vi "Align Trajectory.vi"(4 "Force alignemnt":bool=TRUE, 6 "Indicator":refnum<vi>, 7 "Calibration":T1, 8 "error in":errorcluster, 9 "Tip Coordinates":refnum<vi>, 10 "Target Coordinates":refnum<vi>, 11 "Manipulator Interface":T2) -> (0 "error out":errorcluster, 2 "Error":bool)   [LabVIEW 2012, in "Targeting Unit.lvlib"]
uses:
  Targeting Unit.lvlib
  <vilib>/Analysis/Matrix/Datatypes/RealMatrix.ctl
  <vilib>/Analysis/Matrix/NI_Matrix.lvlib
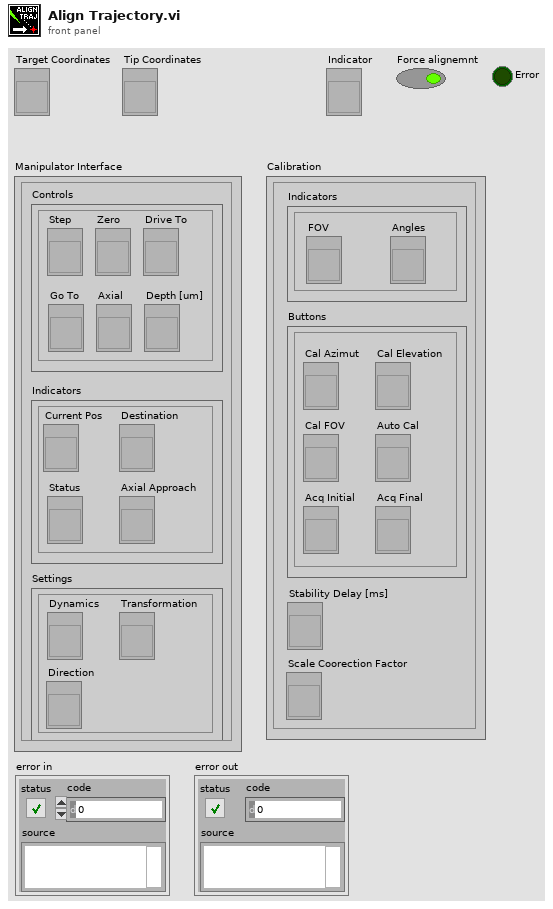
[diagram p1: front panel]
types:
  T1 = cluster{"Indicators":cluster{"FOV":refnum<vi>, "Angles":refnum<vi>}, "Buttons":cluster{"Cal FOV":refnum<vi>, "Cal Azimut":refnum<vi>, "Cal Elevation":refnum<vi>, "Auto Cal":refnum<vi>, "Acq Initial":refnum<vi>, "Acq Final":refnum<vi>}, "Stability Delay [ms]":refnum<vi>, "Scale Coorection Factor":refnum<vi>}
  T2 = cluster{"Indicators":cluster{"Current Pos":refnum<vi>, "Destination":refnum<vi>, "Status":refnum<vi>, "Axial Approach":refnum<vi>}, "Settings":cluster{"Dynamics":refnum<vi>, "Transformation":refnum<vi>, "Direction":refnum<vi>}, "Controls":cluster{"Zero":refnum<vi>, "Step":refnum<vi>, "Drive To":refnum<vi>, "Go To":refnum<vi>, "Axial":refnum<vi>, "Depth [um]":refnum<vi>}}
  T3 = cluster{"X [um]":dbl, "Y [um]":dbl, "Z [um]":dbl}
  T4 = typedef "NI_Matrix.lvlib/RealMatrix.ctl" = dbl[][]
  T5 = cluster{"Step length [um]":dbl, "Interstep Interval [ms]":u32, "Initial Speed [um/s]":dbl, "Max Speed [um/s]":dbl, "Acceleration [um/s^2]":dbl, "Max Depth [um]":dbl, "Max Penetration [um]":dbl}
  T6 = cluster{"X [um]":bool, "Y [um]":bool, "Z [um]":bool}
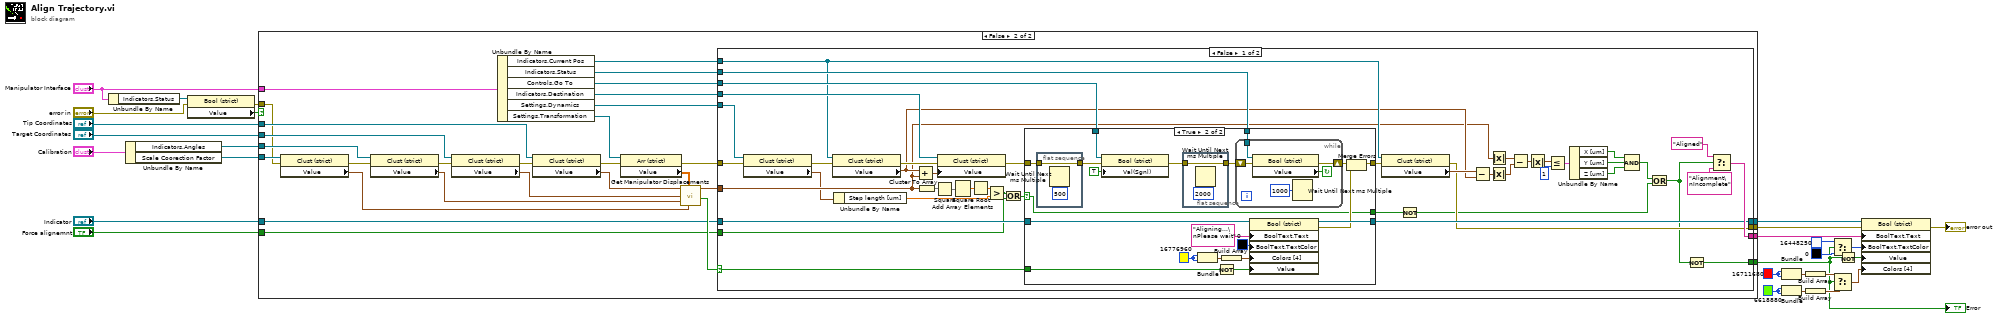
[diagram p0: block diagram]
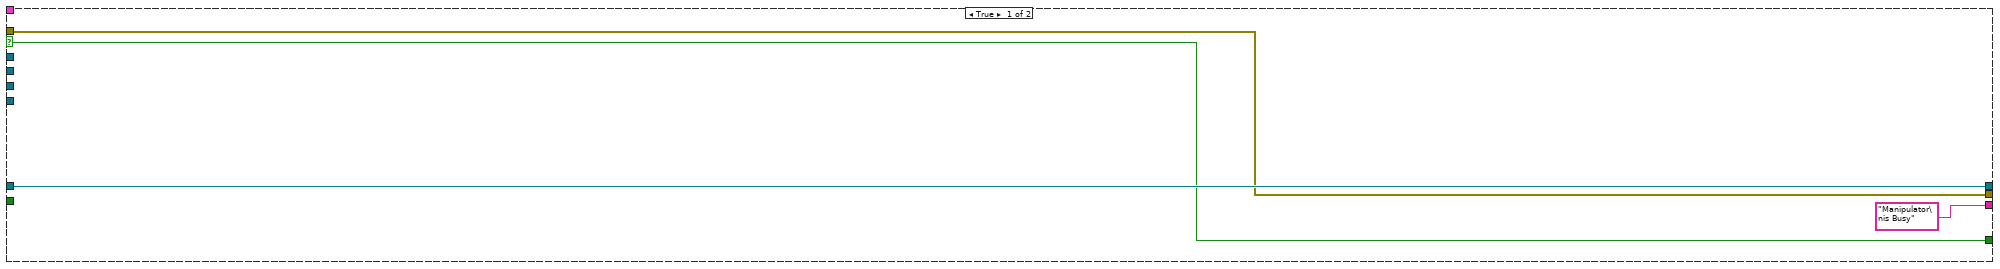
[diagram p2: hidden frame]
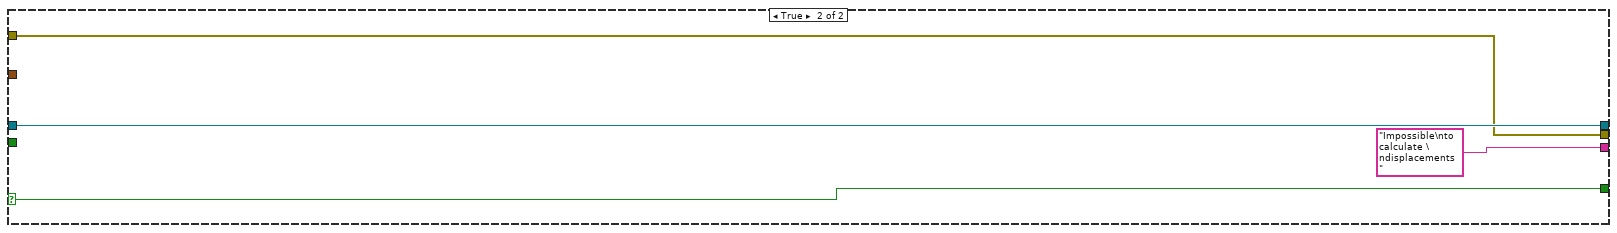
[diagram p4: hidden frame]
diagram:
  w9 = u32 6618880
  w12 = u32 16711680
  n1 = Unbundle By Name("Manipulator Interface") -> ("Indicators.Status"=w17:refnum<vi>)
  n2 = Unbundle By Name("Calibration") -> ("Indicators.Angles"=w3:refnum<vi>, "Scale Coorection Factor"=w2:refnum<vi>)
  n3 = property class="Bool (strict)"(reference=w17, error in="error in") -> (error out=w16:errorcluster, "Value"=w14:bool)  [unwired: 1 out]
  n4 = case shown="False" w14 {
    selector: w14 -> [w30 _]
    tunnel: "Manipulator Interface" -> [_ w62]
    tunnel: "Target Coordinates" -> [_ w61]
    tunnel: "Tip Coordinates" -> [_ w59]
    tunnel: w3 -> [_ w57]
    tunnel: [w31 w49] -> w22
    tunnel: ["Manipulator\nis Busy" ("Window Title (\"\")") w48] -> w21
    tunnel: [w30 w47] -> w5
    tunnel: "Indicator" -> [w32 w46]
    tunnel: [w32 w45] -> w19
    tunnel: w16 -> [w31 w36]
    tunnel: w2 -> [_ w37]
    tunnel: "Force alignemnt" -> [_ w33]
    frame True {
    }
    frame False {
      n5 = property class="Clust (strict)"(reference=w37, error in=w36) -> (error out=w39:errorcluster, "Value"=w38:cluster{"Kx":dbl, "Ky":dbl, "Kz":dbl})  [unwired: 1 out]
      n6 = property class="Clust (strict)"(reference=w57, error in=w39) -> (error out=w43:errorcluster, "Value"=w56:cluster{"Azimut":dbl, "Elevation":dbl})  [unwired: 1 out]
      n7 = property class="Clust (strict)"(reference=w61, error in=w43) -> (error out=w44:errorcluster, "Value"=w60:T3)  [unwired: 1 out]
      n8 = Unbundle By Name(w62) -> ("Indicators.Current Pos"=w50:refnum<vi>, "Indicators.Status"=w51:refnum<vi>, "Controls.Go To"=w52:refnum<vi>, "Indicators.Destination"=w53:refnum<vi>, "Settings.Dynamics"=w34:refnum<vi>, "Settings.Transformation"=w35:refnum<vi>)
      n9 = property class="Clust (strict)"(reference=w59, error in=w44) -> (error out=w42:errorcluster, "Value"=w58:T3)  [unwired: 1 out]
      n10 = property class="Arr (strict)"(reference=w35, error in=w42) -> (error out=w41:errorcluster, "Value"=w55:T4)  [unwired: 1 out]
      n11 = call "Get Manipulator Displacements.vi"("Transformation Matrix"=w55, "Scale Coorection Factor"=w38, "Angles"=w56, "Target Coordinates"=w60, "Tip Coordinates"=w58) -> ("Error"=w54:bool, "Manipulator Displacements"=w40:T3)  [unwired: 4 in, 1 out]
      n12 = case shown="False" w54 {
        selector: w54 -> [w86 w141]
        tunnel: w53 -> [w107 _]
        tunnel: w52 -> [w106 _]
        tunnel: [w82 w141] -> w47
        tunnel: w51 -> [w105 _]
        tunnel: w50 -> [w85 _]
        tunnel: [w75 w140] -> w49
        tunnel: [w89 "Impossible\nto calculate \ndisplacements " ("Window Title (\"\")")] -> w48
        tunnel: w46 -> [w88 w142]
        tunnel: [w87 w142] -> w45
        tunnel: w41 -> [w74 w140]
        tunnel: w40 -> [w77 _]
        tunnel: w34 -> [w72 _]
        tunnel: w33 -> [w68 _]
        frame False {
          n13 = property class="Clust (strict)"(reference=w72, error in=w74) -> (error out=w73:errorcluster, "Value"=w71:T5)  [unwired: 1 out]
          n14 = property class="Clust (strict)"(reference=w85, error in=w73) -> (error out=w96:errorcluster, "Value"=w83:T3)  [unwired: 1 out]
          n15 = Unbundle By Name(w71) -> ("Step length [um]"=w67:dbl)
          n16 = Add(x=w83, y=w77) -> (x+y=w84:T3)
          n17 = Cluster To Array(cluster=w77) -> (array=w78:dbl[])
          n18 = Square(x=w78) -> (x^2=w79:dbl[])
          n19 = property class="Clust (strict)"(reference=w107, error in=w96, "Value"=w84) -> (error out=w81:errorcluster)  [unwired: 1 out]
          n20 = Add Array Elements(numeric array=w79) -> (sum=w80:dbl)
          n21 = Square Root(x=w80) -> (sqrt(x)=w76:dbl)
          n22 = Greater?(x=w76, y=w67) -> (0:w70:bool)
          n23 = Or(x=w70, y=w68) -> (x .or. y?=w69:bool)
          n24 = case shown="True" w69 {
            selector: w69 -> [w108 w111]
            tunnel: w106 -> [_ w129]
            tunnel: w105 -> [_ w128]
            tunnel: [w109 w113] -> w104
            tunnel: w88 -> [w110 w126]
            tunnel: [w110 w125] -> w87
            tunnel: w86 -> [_ w124]
            tunnel: w81 -> [w109 w119]
            tunnel: [w108 w111] -> w64
            frame False {
            }
            frame True {
              w122 = u32 16776960
              n25 = flat-sequence {
                tunnel: [w132] -> w115
                tunnel: w119 -> [w132]
                frame #0 {
                  n26 = Wait Until Next ms Multiple(millisecond multiple=u32 500) -> ()  [unwired: 1 out]
                }
              }
              n27 = property class="Bool (strict)"(reference=w129, error in=w115, "Val(Sgnl)"=TRUE ("Value")) -> (error out=w116:errorcluster)  [unwired: 1 out]
              n28 = flat-sequence {
                tunnel: [w134] -> w117
                tunnel: w116 -> [w134]
                frame #0 {
                  n29 = Wait Until Next ms Multiple(millisecond multiple=u32 2000) -> ()  [unwired: 1 out]
                }
              }
              n30 = Bundle(w122, w122) -> (w121:cluster{u32, u32})  [unwired: 1 in]
              n31 = Not(x=w124) -> (.not. x?=w123:bool)
              n32 = Build Array(w121) -> (w120:cluster{u32, u32}[])
              n33 = while {
                tunnel: w128 -> [w135]
                shift-right: [w136] -> w114
                shift-left: w117 -> [w137]
                stop <- w139 continue-if-true
                n34 = property class="Bool (strict)"(reference=w135, error in=w137) -> (error out=w136:errorcluster, "Value"=w139:bool)  [unwired: 1 out]
                n35 = Wait Until Next ms Multiple(millisecond multiple=u32 1000) -> ()  [unwired: 1 out]
              }
              n36 = property class="Bool (strict)"(reference=w126, "BoolText.Text"="Aligning...\nPlease wait" ("Window Title (\"\")"), "BoolText.TextColor"=u32 0, "Colors [4]"=w120, "Value"=w123) -> (reference out=w125:refnum<vi>, error out=w112:errorcluster)  [unwired: 1 in]
              n37 = Merge Errors(w114, w112) -> (w113:errorcluster)
            }
          }
          n38 = property class="Clust (strict)"(reference=w85, error in=w104) -> (error out=w75:errorcluster, "Value"=w97:T3)  [unwired: 1 out]
          n39 = Not(x=w64) -> (.not. x?=w63:bool)
          n40 = Subtract(x=w97, y=w83) -> (x-y=w103:T3)
          n41 = Absolute Value(x=w77) -> (abs(x)=w98:T3)
          n42 = Absolute Value(x=w103) -> (abs(x)=w100:T3)
          n43 = Subtract(x=w98, y=w100) -> (x-y=w99:T3)
          n44 = Absolute Value(x=w99) -> (abs(x)=w101:T3)
          n45 = Less Or Equal?(x=w101, y=1 ("Y")) -> (x <= y?=w95:T6)
          n46 = Unbundle By Name(w95) -> ("X [um]"=w92:bool, "Y [um]"=w91:bool, "Z [um]"=w90:bool)
          n47 = Compound Arithmetic op=AND(w92, w91, w90) -> (w66:bool)
          n48 = Or(x=w66, y=w63) -> (x .or. y?=w65:bool)
          n49 = Not(x=w65) -> (.not. x?=w82:bool)
          n50 = Select(t="Aligned", s=w65, f="Alignment\nIncomplete" ("Window Title (\"\")")) -> (s? t:f=w89:string)
        }
        frame True {
        }
      }
    }
  }
  "Error" <- w5
  n51 = Bundle(w12, w12) -> (w11:cluster{u32, u32})  [unwired: 1 in]
  n52 = Bundle(w9, w9) -> (w8:cluster{u32, u32})  [unwired: 1 in]
  n53 = Build Array(w11) -> (w10:cluster{u32, u32}[])
  n54 = Build Array(w8) -> (w7:cluster{u32, u32}[])
  n55 = Select(t=u32 16448250, s=w5, f=u32 0) -> (s? t:f=w24:u32)
  n56 = Select(t=w10, s=w5, f=w7) -> (s? t:f=w6:cluster{u32, u32}[])
  n57 = Not(x=w5) -> (.not. x?=w13:bool)
  n58 = property class="Bool (strict)"(reference=w19, error in=w22, "BoolText.Text"=w21, "BoolText.TextColor"=w24, "Value"=w13, "Colors [4]"=w6) -> (error out=→"error out":errorcluster)  [unwired: 1 out]
